vi "Turn.vi"(10 "mode":i32, 11 "Effort":dbl) -> ()   [LabVIEW 2016]
uses:
  <vilib>/Rock Robotics/WPI/SafetyOutput/WPI_SafetyOutputConfigMenu.ctl
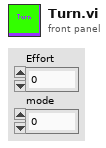
[diagram p1: front panel]
types:
  T1 = typedef "WPI_SafetyOutputConfigMenu.ctl" = enum16{"Enable", "Disable"}
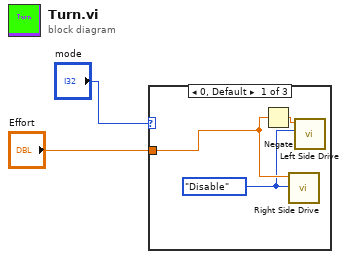
[diagram p0: block diagram]
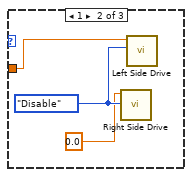
[diagram p2: hidden frame]
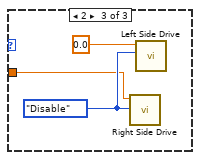
[diagram p3: hidden frame]
diagram:
  n1 = case shown="0, Default" "mode" {
    tunnel: "Effort" -> [w4 w6 w9]
    frame 0, Default {
      w3 = WPI_SafetyOutputConfigMenu."Disable" ("mode")
      n2 = Negate(x=w4) -> (-x=w5:dbl)
      n3 = call "Right Side Drive.vi"("mode"=w3, "Effort"=w4) -> ()  [unwired: 10 in]
      n4 = call "Left Side Drive.vi"("mode"=w3, "Effort"=w5) -> ()  [unwired: 10 in]
    }
    frame 1 {
      w8 = WPI_SafetyOutputConfigMenu."Disable" ("mode")
      n5 = call "Right Side Drive.vi"("mode"=w8, "Effort"=0.0) -> ()  [unwired: 10 in]
      n6 = call "Left Side Drive.vi"("mode"=w8, "Effort"=w6) -> ()  [unwired: 10 in]
    }
    frame 2 {
      w11 = WPI_SafetyOutputConfigMenu."Disable" ("mode")
      n7 = call "Right Side Drive.vi"("mode"=w11, "Effort"=w9) -> ()  [unwired: 10 in]
      n8 = call "Left Side Drive.vi"("mode"=w11, "Effort"=0.0) -> ()  [unwired: 10 in]
    }
  }
